vi "DIO Autonomous Setting Reader.vi"() -> (3 "Numeric":u32)   [LabVIEW 2019]
uses:
  <vilib>/Rock Robotics/Network Tables/NT Write Number.vi
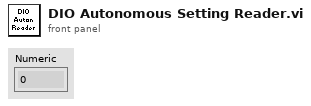
[diagram p1: front panel]
types:
  T1 = typedef "WPI_DigitalInputDevRef.ctl" = cluster{"DevStatus":errorcluster, "DIO Channel":T2}
  T2 = typedef "FPGA_DIOChannel.ctl" = enum8{"DIO 0", "DIO 1", "DIO 2", "DIO 3", "DIO 4", "DIO 5", "DIO 6", "DIO 7", "DIO 8", "DIO 9", "DIO MXP 0", "DIO MXP 1", "DIO MXP 2", "DIO MXP 3", "DIO MXP 4", "DIO MXP 5", "DIO MXP 6", "DIO MXP 7", "DIO MXP 8", "DIO MXP 9", "DIO MXP 10", "DIO MXP 11", "DIO MXP 12", "DIO MXP 13", "DIO MXP 14", "DIO MXP 15", "SPI Port CS1", "SPI Port CS2", "SPI Port CS3", "SPI Port MISO", "SPI Port MOSI", "Invalid"}
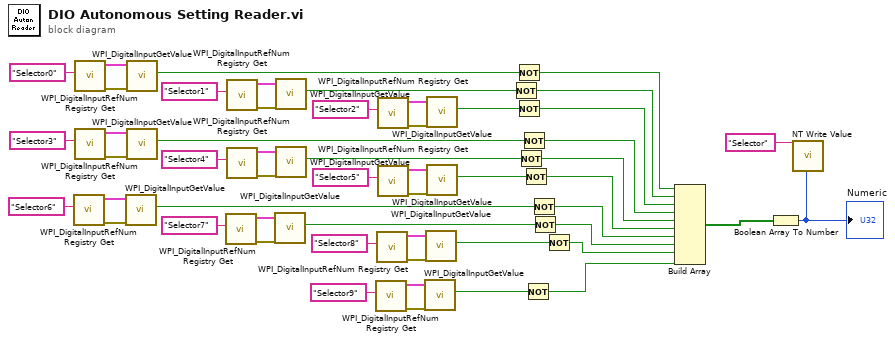
[diagram p0: block diagram]
diagram:
  n1 = call <vilib>:"WPI_DigitalInputRefNum Registry Get.vi"("refnum name"="Selector6") -> ("error out"=w38:errorcluster, "DigitalInputDevRef"=w37:T1)  [unwired: 9 in]
  n2 = call <vilib>:"WPI_DigitalInputRefNum Registry Get.vi"("refnum name"="Selector0") -> ("error out"=w16:errorcluster, "DigitalInputDevRef"=w15:T1)  [unwired: 9 in]
  n3 = call <vilib>:"WPI_DigitalInputRefNum Registry Get.vi"("refnum name"="Selector3") -> ("error out"=w26:errorcluster, "DigitalInputDevRef"=w25:T1)  [unwired: 9 in]
  n4 = call <vilib>:"WPI_DigitalInputGetValue.vi"("error in (no error)"=w38, "DigitalInputDevRef"=w37) -> ("Value"=w43:bool)  [unwired: 7 in, 2 out]
  n5 = call <vilib>:"WPI_DigitalInputGetValue.vi"("error in (no error)"=w16, "DigitalInputDevRef"=w15) -> ("Value"=w47:bool)  [unwired: 7 in, 2 out]
  n6 = call <vilib>:"WPI_DigitalInputGetValue.vi"("error in (no error)"=w26, "DigitalInputDevRef"=w25) -> ("Value"=w31:bool)  [unwired: 7 in, 2 out]
  n7 = call <vilib>:"WPI_DigitalInputRefNum Registry Get.vi"("refnum name"="Selector7") -> ("error out"=w34:errorcluster, "DigitalInputDevRef"=w35:T1)  [unwired: 9 in]
  n8 = call <vilib>:"WPI_DigitalInputRefNum Registry Get.vi"("refnum name"="Selector1") -> ("error out"=w12:errorcluster, "DigitalInputDevRef"=w13:T1)  [unwired: 9 in]
  n9 = call <vilib>:"WPI_DigitalInputRefNum Registry Get.vi"("refnum name"="Selector4") -> ("error out"=w22:errorcluster, "DigitalInputDevRef"=w23:T1)  [unwired: 9 in]
  n10 = call <vilib>:"WPI_DigitalInputGetValue.vi"("error in (no error)"=w34, "DigitalInputDevRef"=w35) -> ("Value"=w44:bool)  [unwired: 7 in, 2 out]
  n11 = call <vilib>:"WPI_DigitalInputGetValue.vi"("error in (no error)"=w12, "DigitalInputDevRef"=w13) -> ("Value"=w11:bool)  [unwired: 7 in, 2 out]
  n12 = call <vilib>:"WPI_DigitalInputGetValue.vi"("error in (no error)"=w22, "DigitalInputDevRef"=w23) -> ("Value"=w32:bool)  [unwired: 7 in, 2 out]
  n13 = call <vilib>:"WPI_DigitalInputRefNum Registry Get.vi"("refnum name"="Selector9") -> ("error out"=w50:errorcluster, "DigitalInputDevRef"=w51:T1)  [unwired: 9 in]
  n14 = call <vilib>:"WPI_DigitalInputRefNum Registry Get.vi"("refnum name"="Selector8") -> ("error out"=w40:errorcluster, "DigitalInputDevRef"=w41:T1)  [unwired: 9 in]
  n15 = call <vilib>:"WPI_DigitalInputRefNum Registry Get.vi"("refnum name"="Selector2") -> ("error out"=w18:errorcluster, "DigitalInputDevRef"=w19:T1)  [unwired: 9 in]
  n16 = call <vilib>:"WPI_DigitalInputRefNum Registry Get.vi"("refnum name"="Selector5") -> ("error out"=w28:errorcluster, "DigitalInputDevRef"=w29:T1)  [unwired: 9 in]
  n17 = call <vilib>:"WPI_DigitalInputGetValue.vi"("error in (no error)"=w50, "DigitalInputDevRef"=w51) -> ("Value"=w53:bool)  [unwired: 7 in, 2 out]
  n18 = call <vilib>:"WPI_DigitalInputGetValue.vi"("error in (no error)"=w40, "DigitalInputDevRef"=w41) -> ("Value"=w45:bool)  [unwired: 7 in, 2 out]
  n19 = call <vilib>:"WPI_DigitalInputGetValue.vi"("error in (no error)"=w18, "DigitalInputDevRef"=w19) -> ("Value"=w21:bool)  [unwired: 7 in, 2 out]
  n20 = call <vilib>:"WPI_DigitalInputGetValue.vi"("error in (no error)"=w28, "DigitalInputDevRef"=w29) -> ("Value"=w33:bool)  [unwired: 7 in, 2 out]
  n21 = Not(x=w11) -> (.not. x?=w9:bool)
  n22 = Not(x=w47) -> (.not. x?=w10:bool)
  n23 = Not(x=w21) -> (.not. x?=w8:bool)
  n24 = Not(x=w32) -> (.not. x?=w6:bool)
  n25 = Not(x=w31) -> (.not. x?=w7:bool)
  n26 = Not(x=w33) -> (.not. x?=w5:bool)
  n27 = Not(x=w53) -> (.not. x?=w1:bool)
  n28 = Not(x=w43) -> (.not. x?=w4:bool)
  n29 = Not(x=w44) -> (.not. x?=w3:bool)
  n30 = Not(x=w45) -> (.not. x?=w2:bool)
  n31 = Build Array(w10, w9, w8, w7, w6, w5, w4, w3, w2, w1) -> (w46:bool[])
  n32 = Boolean Array To Number(Boolean array=w46) -> (number=w48:u32)
  "Numeric" <- w48
  n33 = call-poly <vilib>:"NT Write Value.vi"("Numeric"=w48, "Name"="Selector") -> ()  [unwired: 9 in, 1 out]
